vi "myRIO_BRig_RT_dataMTrig_Laser_Tcycle.vi"() -> (2 "output_Laser_Tcycle":i32)   [LabVIEW 2014]
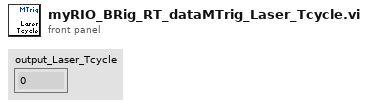
[diagram p1: front panel]
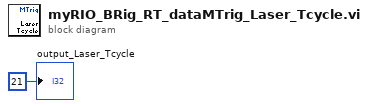
[diagram p0: block diagram]
diagram:
  "output_Laser_Tcycle" <- 21 ("output_iBlock")
